vi "setRampParameters.vi"(8 "error in (no error)":errorcluster, 10 "RampParameters":T1, 11 "RampTone in":refnum<class "RampTone.lvclass">) -> (0 "error out":errorcluster, 3 "RampTone out":refnum<class "RampTone.lvclass">)   [LabVIEW 2011, in "Tools.lvlib" / "Scripting.lvlib" / "RampTone.lvclass"]
uses:
  RampTone.lvclass
  SingleTone/SingleTone.lvclass
  RampTone.lvclass/RampTone.ctl
  ScriptEvent.lvclass
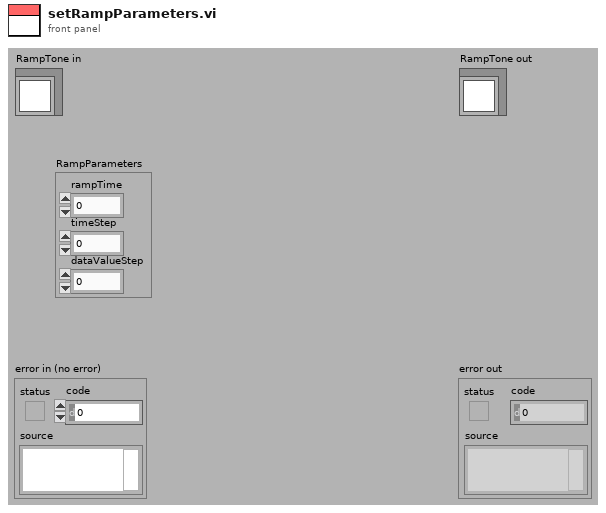
[diagram p1: front panel]
types:
  T1 = cluster{"rampTime":dbl, "timeStep":dbl, "dataValueStep":dbl}
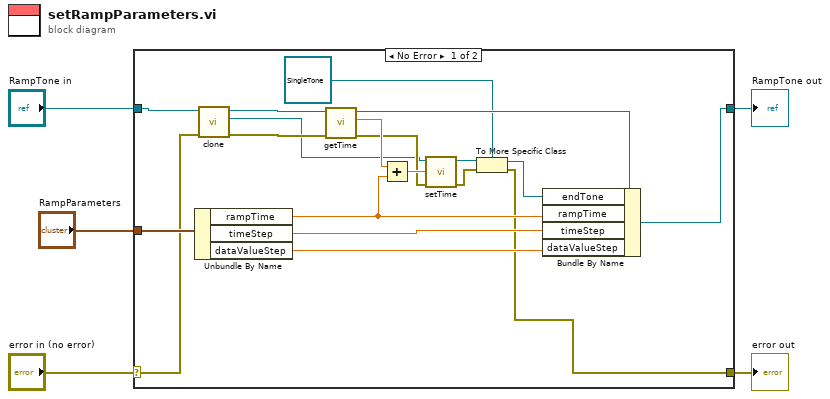
[diagram p0: block diagram]
diagram:
  n1 = case shown="No Error" "error in (no error)" {
    selector: "error in (no error)" -> [w12 w26]
    tunnel: [w6 w26] -> w4
    tunnel: [w21 w25] -> w2
    tunnel: "RampTone in" -> [w15 w25]
    tunnel: "RampParameters" -> [w24 _]
    frame No Error {
      n2 = Unbundle By Name(w24) -> ("rampTime"=w13:dbl, "timeStep"=w23:dbl, "dataValueStep"=w22:dbl)
      n3 = call-dynamic "clone.vi"("error in (no error)"=w12, "SingleTone in"=w15) -> ("error out"=w18:errorcluster, "clone"=w10:refnum<class "ScriptEvent.lvclass">, "SingleTone out"=w17:refnum<class "RampTone.lvclass">)  [unwired: 7 in]
      n4 = call "getTime.vi"("error in (no error)"=w18, "ScriptEvent.lvclass in"=w17) -> ("error out"=w16:errorcluster, "time"=w19:dbl, "ScriptEvent.lvclass out"=w14:refnum<class "RampTone.lvclass">)  [unwired: 7 in]
      n5 = Add(x=w19, y=w13) -> (x+y=w20:dbl)
      n6 = call "setTime.vi"("error in (no error)"=w16, "time"=w20, "ScriptEvent.lvclass in"=w10) -> ("error out"=w7:errorcluster, "ScriptEvent.lvclass out"=w11:refnum<class "ScriptEvent.lvclass">)  [unwired: 7 in]
      n7 = To More Specific Class(target class=refnum<class "SingleTone.lvclass"> refnum ("Tools.lvlib:Scripting.lvlib:SingleTone.lvclass"), reference=w11, error in=w7) -> (specific class reference=w9:refnum<class "SingleTone.lvclass">, error out=w6:errorcluster)
      n8 = Bundle By Name(cluster=w14, "endTone"=w9, "rampTime"=w13, "timeStep"=w23, "dataValueStep"=w22) -> (w21:refnum<class "RampTone.lvclass">)
    }
    frame Error {
    }
  }
  "error out" <- w4
  "RampTone out" <- w2
